vi "ReadWriteLines.vi"() -> ()   [LabVIEW 2015]
uses:
  <vilib>/Utility/error.llb/DialogType.ctl
  <vilib>/DAQmx/read.llb/DAQmx Read (Digital Bool 1Line 1Point).vi
  <vilib>/DAQmx/write.llb/DAQmx Write (Digital 1D Bool 1Chan 1Samp).vi
  <vilib>/DAQmx/create/channels.llb/DAQmx Create Channel (DO-Digital Output).vi
  <vilib>/DAQmx/create/channels.llb/DAQmx Create Channel (DI-Digital Input).vi
  <vilib>/DAQmx/miscellaneous.llb/DAQmx Fill In Error Info.vi
panel:
  out "Dato leido\nen Linea 3":bool
  in  "stop":bool
  in  "data 2":bool[](array[boolean])
  in  "data":bool[](array[boolean])
  in  "lines 3":tag
  in  "lines 2":tag
  in  "lines":tag
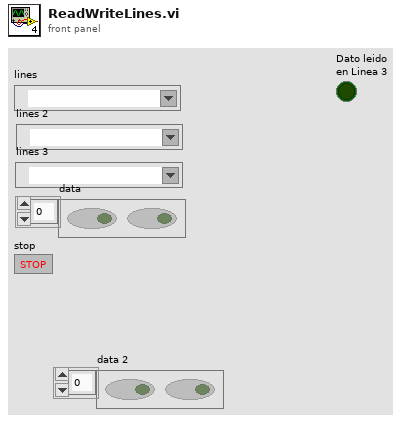
[diagram p1: front panel]
types:
  T1 = typedef "DialogType.ctl" = u16
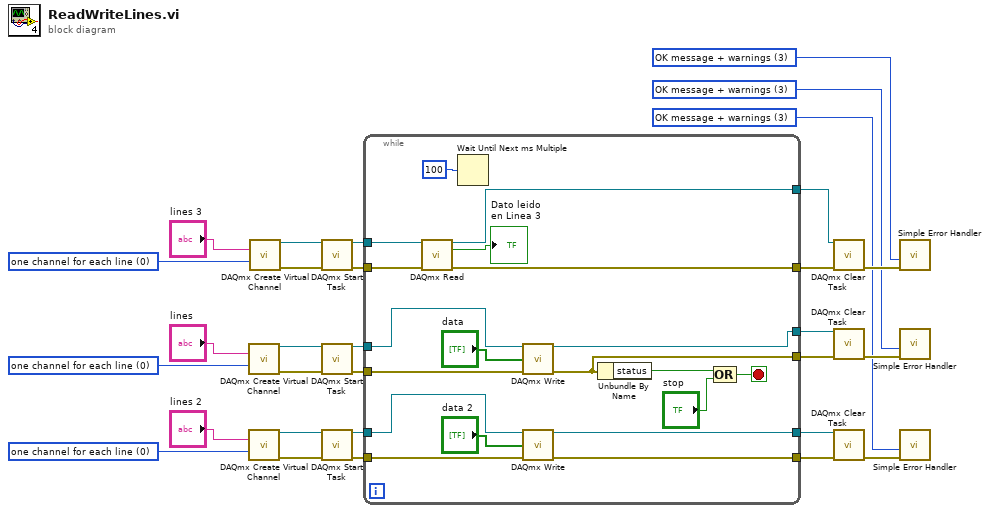
[diagram p0: block diagram]
diagram:
  w1 = T1 3 items=["no dialog", "OK message", "continue or stop message", "OK message + warnings", "continue/stop + warnings"] ("type of dialog (OK msg:1)")
  w2 = T1 3 items=["no dialog", "OK message", "continue or stop message", "OK message + warnings", "continue/stop + warnings"] ("type of dialog (OK msg:1)")
  w3 = T1 3 items=["no dialog", "OK message", "continue or stop message", "OK message + warnings", "continue/stop + warnings"] ("type of dialog (OK msg:1)")
  w25 = 0 items=["one channel for each line", "one channel for all lines"] ("line grouping")
  w26 = 0 items=["one channel for each line", "one channel for all lines"] ("line grouping")
  w27 = 0 items=["one channel for each line", "one channel for all lines"] ("line grouping")
  n1 = call-poly <vilib>:"DAQmx Create Virtual Channel.vi"("lines"="lines", "line grouping"=w27) -> ("task out"=w24:refnum<k21>, "error out"=w23:errorcluster)  [unwired: 12 in]
  n2 = call-poly <vilib>:"DAQmx Create Virtual Channel.vi"("lines"="lines 2", "line grouping"=w26) -> ("task out"=w22:refnum<k21>, "error out"=w21:errorcluster)  [unwired: 12 in]
  n3 = call-poly <vilib>:"DAQmx Create Virtual Channel.vi"("lines"="lines 3", "line grouping"=w25) -> ("task out"=w20:refnum<k21>, "error out"=w19:errorcluster)  [unwired: 12 in]
  n4 = call <vilib>:"DAQmx Start Task.vi"("task/channels in"=w20, "error in"=w19) -> ("task out"=w14:refnum<k21>, "error out"=w13:errorcluster)  [unwired: 12 in]
  n5 = call <vilib>:"DAQmx Start Task.vi"("task/channels in"=w24, "error in"=w23) -> ("task out"=w18:refnum<k21>, "error out"=w17:errorcluster)  [unwired: 12 in]
  n6 = call <vilib>:"DAQmx Start Task.vi"("task/channels in"=w22, "error in"=w21) -> ("task out"=w16:refnum<k21>, "error out"=w15:errorcluster)  [unwired: 12 in]
  n7 = while {
    tunnel: w18 -> [w47]
    tunnel: w17 -> [w46]
    tunnel: w16 -> [w44]
    tunnel: w15 -> [w43]
    tunnel: w14 -> [w42]
    tunnel: w13 -> [w41]
    tunnel: [w40] -> w10
    tunnel: [w35] -> w9
    tunnel: [w39] -> w8
    tunnel: [w38] -> w7
    tunnel: [w37] -> w12
    tunnel: [w36] -> w11
    stop <- w32 stop-if-true
    n8 = call-poly <vilib>:"DAQmx Read.vi"("task/channels in"=w42, "error in"=w41) -> ("task out"=w37:refnum<k21>, "data"=→"Dato leido\nen Linea 3":bool, "error out"=w36:errorcluster)  [unwired: 11 in]
    n9 = Wait Until Next ms Multiple(millisecond multiple=u32 100) -> ()  [unwired: 1 out]
    n10 = call-poly <vilib>:"DAQmx Write.vi"("task/channels in"=w47, "data"="data", "error in"=w46) -> ("task out"=w40:refnum<k21>, "error out"=w35:errorcluster)  [unwired: 10 in, 1 out]
    n11 = call-poly <vilib>:"DAQmx Write.vi"("task/channels in"=w44, "data"="data 2", "error in"=w43) -> ("task out"=w39:refnum<k21>, "error out"=w38:errorcluster)  [unwired: 10 in, 1 out]
    n12 = Unbundle By Name(w35) -> ("status"=w34:bool)
    n13 = Compound Arithmetic op=OR(w34, "stop") -> (w32:bool)
  }
  n14 = call <vilib>:"DAQmx Clear Task.vi"("task in"=w12, "error in"=w11) -> ("error out"=w4:errorcluster)  [unwired: 13 in]
  n15 = call <vilib>:"DAQmx Clear Task.vi"("task in"=w10, "error in"=w9) -> ("error out"=w5:errorcluster)  [unwired: 13 in]
  n16 = call <vilib>:"DAQmx Clear Task.vi"("task in"=w8, "error in"=w7) -> ("error out"=w6:errorcluster)  [unwired: 13 in]
  n17 = call <vilib>:"Simple Error Handler.vi"("type of dialog (OK msg:1)"=w1, "error in (no error)"=w4) -> ()  [unwired: 3 in, 5 out]
  n18 = call <vilib>:"Simple Error Handler.vi"("type of dialog (OK msg:1)"=w2, "error in (no error)"=w5) -> ()  [unwired: 3 in, 5 out]
  n19 = call <vilib>:"Simple Error Handler.vi"("type of dialog (OK msg:1)"=w3, "error in (no error)"=w6) -> ()  [unwired: 3 in, 5 out]
